vi "Handle Command.vi"(7 "Communication References":T2={"BCI-1553-RSP"="BCI-1553-RSP", "BCI-1553-CMD"="BCI-1553-CMD"}, 10 "BCI-1553 References":T1) -> ()   [LabVIEW 2020, in "BCI-1553 RT Interface.lvlib"]
doc: "Reads and handles commands from the RealTime API. Commands are parsed and then distributed to the appropriate module."
uses:
  BCI-1553 RT Interface.lvlib
  Public/Type Defs/Communication References.ctl
  Public/Type Defs/BCI-1553 References.ctl
  <vilib>/rvi/DataTransferAndStorage/Container/Common/niFpgaContainerExecOnDevCompGetState.vi
  <vilib>/rvi/Emulation/niFpgaEmulationIsFPGAContextNoSignature.vi
  <vilib>/rvi/Emulation/niFpgaSctlEmulationGetInTimedLoop.vi
  <vilib>/rvi/errors/niFpgaSetErrorForExecOnDevCompSimple.vi
  <vilib>/rvi/eio/common/nirviEmuReportErrorAndStop.vi
  <vilib>/rvi/DataTransferAndStorage/Container/Common/niFpgaContainerGetUniqueNameForEmu.vi
  <vilib>/rvi/FIFO/Fifo_Resource/nirvififoEmulationSetSize.vi
  <vilib>/rvi/FIFO/Fifo_Resource/nirviFifoEmulationQueueMgr.vi
  <instcachedir>/0/nirviFifoEmulationQueueMgr_E5CAEC123FF24DC58D834DCA3CDAA9B5.lvgen/nirviFifoEmulationQueueMgr_E5CAEC123FF24DC58D834DCA3CDAA9B5_001.vi
  <vilib>/rvi/FIFO/Fifo_Resource/nirvififoEmulationDetermineInputValidOut.vi
  <vilib>/rvi/FIFO/Fifo_Resource/nirvififoEmulationCreateLock.vi
  <vilib>/rvi/Emulation/niFpgaProcessEmulError.vi
  <vilib>/rvi/FIFO/Fifo_Resource/nirvififoEmulationObtainLock.vi
  <vilib>/rvi/FIFO/Fifo_Resource/nirvififoEmulationReleaseLock.vi
  <vilib>/rvi/occurrence/nirviWaitOnOccurrenceBase.vi
  <vilib>/rvi/errors/nirviReportUnexpectedCaseInternalError.vi
  <vilib>/rvi/errors/nirviReportUnexpectedCaseInternalError (U32).vi
  <vilib>/Utility/error.llb/Clear Errors.vi
  <vilib>/rvi/interface/RandomDataEmulation/niFpgaRandomDataHandleErrors.vi
  <vilib>/rvi/DataTransferAndStorage/Container/XNode/niFpgaContainer.xnode
  <vilib>/rvi/FIFO/Fifo_Resource/niFpgaFifoEmulationRefIn.vi
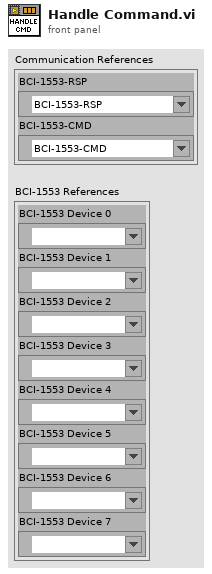
[diagram p1: front panel]
types:
  T1 = typedef "BCI-1553 RT Interface.lvlib/BCI-1553 References.ctl" = cluster{"BCI-1553 Device 0":refnum<k21>, "BCI-1553 Device 1":refnum<k21>, "BCI-1553 Device 2":refnum<k21>, "BCI-1553 Device 3":refnum<k21>, "BCI-1553 Device 4":refnum<k21>, "BCI-1553 Device 5":refnum<k21>, "BCI-1553 Device 6":refnum<k21>, "BCI-1553 Device 7":refnum<k21>}
  T2 = typedef "BCI-1553 RT Interface.lvlib/Communication References.ctl" = cluster{"BCI-1553-RSP":refnum<k21>, "BCI-1553-CMD":refnum<k21>}
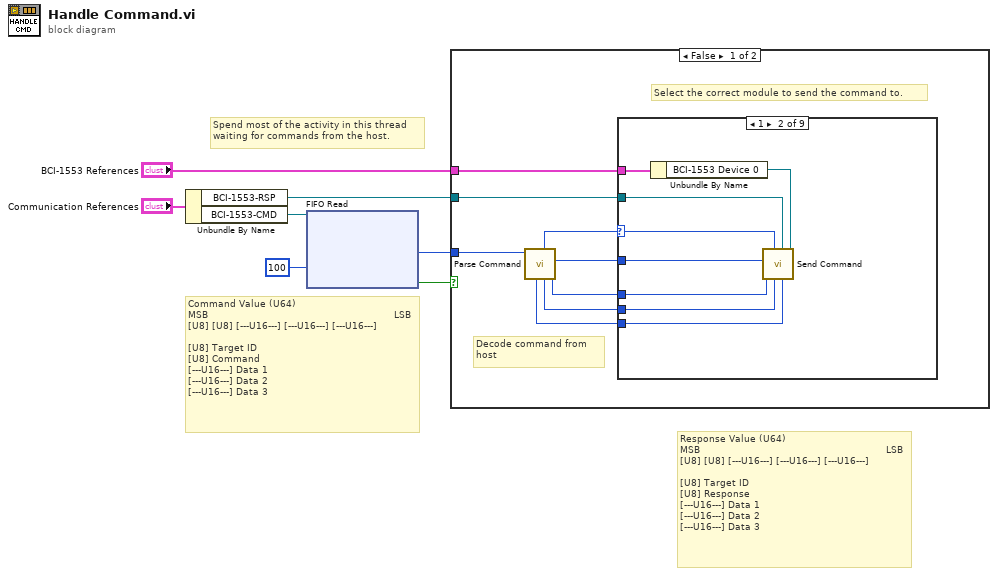
[diagram p0: block diagram]
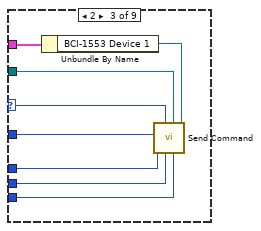
[diagram p3: hidden frame]
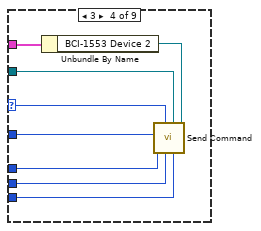
[diagram p4: hidden frame]
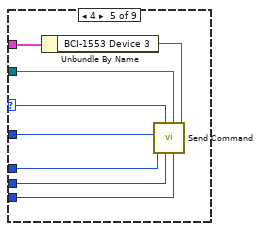
[diagram p5: hidden frame]
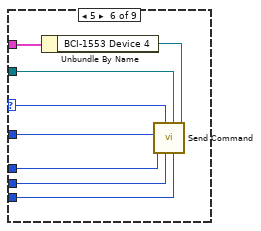
[diagram p6: hidden frame]
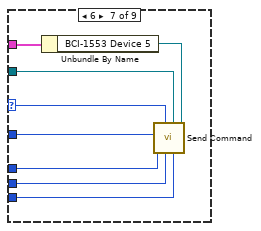
[diagram p7: hidden frame]
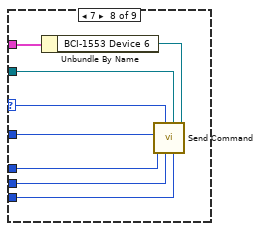
[diagram p8: hidden frame]
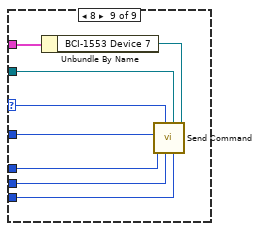
[diagram p9: hidden frame]
diagram:
  # "Spend most of the activity in this thread\nwaiting for commands from the host."
  # "Response Value (U64)\nMSB                                                              LSB\n[U8] [U8] [---U16---] [---U16---] [---U16---]\n\n[U8] Target ID\n[U8] Response\n[---U16---] Data 1\n[---U16---] Data 2\n[---U16---] Data 3"
  # "Command Value (U64)\nMSB                                                              LSB\n[U8] [U8] [---U16---] [---U16---] [---U16---]\n\n[U8] Target ID\n[U8] Command\n[---U16---] Data 1\n[---U16---] Data 2\n[---U16---] Data 3"
  n1 = Unbundle By Name("Communication References") -> ("BCI-1553-RSP"=w2:refnum<k21>, "BCI-1553-CMD"=w3:refnum<k21>)
  n2 = xnode ("FIFO Read")("Timeout"=100, "FIFO In"=w3) -> ("Element"=w5:u64, "Timed Out?"=w6:bool)  [unwired: 1 out]
  n3 = case shown="False" w6 {
    tunnel: w5 -> [w15 _]
    tunnel: w2 -> [w8 _]
    tunnel: "BCI-1553 References" -> [w14 _]
    frame False {
      # "Select the correct module to send the command to."
      # "Decode command from\nhost"
      n4 = call "Parse Command.vi"("Command"=w15) -> ("Data 1"=w13:u16, "Command"=w9:u8, "Data 2"=w12:u16, "Target ID"=w10:u8, "Data 3"=w11:u16)  [unwired: 6 in]
      n5 = case shown="1" w10 {
        selector: w10 -> [_ w16 w24 w32 w40 w48 w56 w64 w72]
        tunnel: w14 -> [_ w23 w31 w39 w47 w55 w63 w71 w79]
        tunnel: w13 -> [_ w21 w29 w37 w45 w53 w61 w69 w77]
        tunnel: w12 -> [_ w20 w28 w36 w44 w52 w60 w68 w76]
        tunnel: w11 -> [_ w19 w27 w35 w43 w51 w59 w67 w75]
        tunnel: w9 -> [_ w22 w30 w38 w46 w54 w62 w70 w78]
        tunnel: w8 -> [_ w17 w25 w33 w41 w49 w57 w65 w73]
        frame Default {
        }
        frame 1 {
          n6 = Unbundle By Name(w23) -> ("BCI-1553 Device 0"=w18:refnum<k21>)
          n7 = call "Send Command.vi"("BCI-1553 Device"=w18, "Data 3"=w19, "BCI-1553-RSP"=w17, "Data 2"=w20, "Target ID"=w16, "Data 1"=w21, "Command"=w22) -> ()  [unwired: 5 in]
        }
        frame 2 {
          n8 = Unbundle By Name(w31) -> ("BCI-1553 Device 1"=w26:refnum<k21>)
          n9 = call "Send Command.vi"("BCI-1553 Device"=w26, "Data 3"=w27, "BCI-1553-RSP"=w25, "Data 2"=w28, "Target ID"=w24, "Data 1"=w29, "Command"=w30) -> ()  [unwired: 5 in]
        }
        frame 3 {
          n10 = Unbundle By Name(w39) -> ("BCI-1553 Device 2"=w34:refnum<k21>)
          n11 = call "Send Command.vi"("BCI-1553 Device"=w34, "Data 3"=w35, "BCI-1553-RSP"=w33, "Data 2"=w36, "Target ID"=w32, "Data 1"=w37, "Command"=w38) -> ()  [unwired: 5 in]
        }
        frame 4 {
          n12 = Unbundle By Name(w47) -> ("BCI-1553 Device 3"=w42:refnum<k21>)
          n13 = call "Send Command.vi"("BCI-1553 Device"=w42, "Data 3"=w43, "BCI-1553-RSP"=w41, "Data 2"=w44, "Target ID"=w40, "Data 1"=w45, "Command"=w46) -> ()  [unwired: 5 in]
        }
        frame 5 {
          n14 = Unbundle By Name(w55) -> ("BCI-1553 Device 4"=w50:refnum<k21>)
          n15 = call "Send Command.vi"("BCI-1553 Device"=w50, "Data 3"=w51, "BCI-1553-RSP"=w49, "Data 2"=w52, "Target ID"=w48, "Data 1"=w53, "Command"=w54) -> ()  [unwired: 5 in]
        }
        frame 6 {
          n16 = Unbundle By Name(w63) -> ("BCI-1553 Device 5"=w58:refnum<k21>)
          n17 = call "Send Command.vi"("BCI-1553 Device"=w58, "Data 3"=w59, "BCI-1553-RSP"=w57, "Data 2"=w60, "Target ID"=w56, "Data 1"=w61, "Command"=w62) -> ()  [unwired: 5 in]
        }
        frame 7 {
          n18 = Unbundle By Name(w71) -> ("BCI-1553 Device 6"=w66:refnum<k21>)
          n19 = call "Send Command.vi"("BCI-1553 Device"=w66, "Data 3"=w67, "BCI-1553-RSP"=w65, "Data 2"=w68, "Target ID"=w64, "Data 1"=w69, "Command"=w70) -> ()  [unwired: 5 in]
        }
        frame 8 {
          n20 = Unbundle By Name(w79) -> ("BCI-1553 Device 7"=w74:refnum<k21>)
          n21 = call "Send Command.vi"("BCI-1553 Device"=w74, "Data 3"=w75, "BCI-1553-RSP"=w73, "Data 2"=w76, "Target ID"=w72, "Data 1"=w77, "Command"=w78) -> ()  [unwired: 5 in]
        }
      }
    }
    frame True {
    }
  }
